vi "FITS - Make Single FITS Header.vi"(7 "Neo Info":T1={"Handle"=104, "Pixel Encoding"="Mono16", "AOI Width"=2560, "AOI Height"=2160, "AOI Stride"=5136, "Image Bytes"=11098896, "Image Pixels"=5529600, "Row Readout Time"=9.371428571428572e-06, "Frame Readout Time"=0.010121142857142858, "Interframe Time"=8.434285714285715e-05, "Semaphore"=refnum, "SerialNumber"="SCC-02209", "Camera Model"="DC-152Q-C00-FI", "Controller ID"="3", "Firmware Version"="13.8.26.122", "Shutter"="Global", "Binning"=0, "Time at Synch"=timestamp(3029526000.379448 s since 1904-01-01), "Idx"=0} {"Time at Synch" format="%<%H:%M:%S>T"; "Interframe Time" format="%#_3g"; "Frame Readout Time" format="%_3g"; "Row Readout Time" format="%_3g"}, 8 "error in":errorcluster, 9 "NAXIS":string="2", 10 "FITS Header":T3={"Wavelength (nm)"=530.15, "Exposure (s)"=0.05, "Tuning Delay (ms)"=1000.0, "Beam Type (-1/1)"=1.0, "Tuning Voltages"=[1.111, 2.222, 3.333, 4.444], "Observer"="observer", "Light Shapping Diffuser"=enum."In Beam", "Comment"="", "Data Type"=9, "Mod Cycles"=0, "SCD Calibration Optics"=enum."1 - Polarizer @0, I+Q", "SCD Emission Line Filter"=enum."1-557.6nm", "Cookbook"="", "COMP-S Calibration Wheel"=enum."Dark", "COMP-S Andover Filter Wheel"=enum."530.3nm/HWB 0.34nm (Fe XIV)", "FOV Rotation (deg)"=66.0, "Objective Lens Position (mm)"=0.0, "Occulter size"=0.0, "Time End"=timestamp(3382374145.421875 s since 1904-01-01), "Acc Exposure (s)"=0.0, "Time Stamp Array"=[], "Camera Serial Number"=[], "Camera Temp"=[], "Camera PI (mm)"=[0.0, 0.0, 0.0], "Time Start"=timestamp(3382374145.421875 s since 1904-01-01), "Peripherals"={"ILX controler"=FALSE, "Zone temperatures"=FALSE, "Andor"=FALSE, "Andor 2"=FALSE, "PI Stages"=FALSE, "AISAS mechanisms"=FALSE, "AISAS Mech.lvclass"=refnum, "Zone temp ref"=variant, "FWs"=FALSE}, "FITS paths"=[path " ", path " ", path " ", path " "], "Cameras"=enum."Andor", "load preset cbk"=FALSE, "periodic check count"=0} {"Camera PI (mm)" format="%_3g"; "Acc Exposure (s)" format="%^.3g"; "Occulter size" format="%.2f"; "Objective Lens Position (mm)" min=70.0 max=152.0 format="%.2f"; "FOV Rotation (deg)" format="%.1f"; "Data Type" items=["LIVE", "DARK", "FLAT", "CALI", "OBSE", "ABSO", "AURE", "TARG", "OBJE", "HOLE", "OREX", "THRO", "CHIP"]; "Exposure (s)" format="%^.3g"; "Wavelength (nm)" format="%_6g"}, 11 "Image #":i32) -> (0 "error out":errorcluster, 1 "23040 Byte Header":string="SIMPLE  =                              T / CONFORMS TO FITS STANDARD            BITPIX  =                             32 / BITS PER PIXEL                       NAXIS   =                              2 / DATA DIMENSIONS IN FITS FILE         NAXIS1  =                              0 / XDIM (PIXELS)                        NAXIS2  =                              0 / YDIM (PIXELS)                        NAXIS3  =                              4 / 4 POLARIZATION STATES                NAXIS4  =                              1 / 1 CAMERA                             ORIGIN  =                        'AISAS' / SCIENTIFIC GROUP                     OBSERVER=                     'SCHWARTZ' / NAME OF OBSERVER                     TELESCOP=                   '20CM ZEISS' / NAME OF TELESCOPE                    LOCATION=            'LOMNICKY PEAK OBS' / LOCATION OF TELESCOPE                INSTRUME=                          'SCD' / NAME OF INSTRUMENT                   BZERO   =                             0. /  ADU OFFSET                          FOCUS   =                             26 / CAMERA-STAGE POSITION (MM)           ROTPOS  =                           66.0 / ROTATIONAL POSITION (DEG)            DIFFUSER=                      'IN BEAM' / 0=IN BEAM, 1=OUT OF BEAM             FW-WVLNG=                        '557.6' / PRE-FILTER CENTER WAVELENGTH (NM)    FW-CALIB=                         'DARK' / CAL-WHEEL POSITION                   CAM-SN1 =                    'SCC-02209' / CAMERA SERIAL NUMBER                 CAM-TEMP=                       0.000000 / FOCAL PLANE TEMP (C)                 TUNEDLAY=                           1000 / LCVR RELAXATION DELAY (mS)           DATE_OBS=                     '3/7/2011' / DATE OF OBSERVATION START (UTC)      TIME_OBS=                   '212225.421' / TIME OF OBSERVATION (UTC)            EXPOSURE=                       0.050000 / EXPOSURE TIME (S)                    MODC    =                              0 / NUMBER OF IMAGES AT EACH STATE       NLC-1   =                          1.111 / TUNING VOLTAGE-1                     NLC-2   =                          2.222 / TUNING VOLTAGE-2                     NLC-3   =                          3.333 / TUNING VOLTAGE-3                     NLC-4   =                          4.444 / TUNING VOLTAGE-4                     NLC-5   =                          0.000 / TUNING VOLTAGE-5                     BEAM    =                              1 / BEAM (0=ON BAND OR 1=CONTINUUM)      WAVELENG=                         530.15 / WAVELENGTH OF OBS (NM)               COMMHEAD=                             '' / OBSERVER COMMENT                     COOKBOOK=                                / COOKBOOK  LOADED                     COMMENT                                                                         COMMENT                                                                         COMMENT                                                                         COMMENT                                                                         COMMENT                                                                         COMMENT                                                                         COMMENT                                                                         COMMENT                                                                         COMMENT                                                                         COMMENT                                                                         COMMENT                                                                         COMMENT                                                                         COMMENT                                                                         COMMENT                                                                         COMMENT                                                                         COMMENT                                                                         COMMENT                                                                         COMMENT                                                                         COMMENT                                                                         COMMENT                                                                         COMMENT                                                                         COMMENT                                                                         COMMENT                                                                         COMMENT                                                                         COMMENT                                                                         COMMENT                                                                         COMMENT                                                                         COMMENT                                                                         COMMENT                                                                         COMMENT                                                                         COMMENT                                                                         COMMENT                                                                         COMMENT                                                                         COMMENT                                                                         COMMENT                                                                         COMMENT                                                                         COMMENT                                                                         COMMENT                                                                         COMMENT                                                                         COMMENT                                                                         COMMENT                                                                         COMMENT                                                                         COMMENT                                                                         COMMENT                                                                         COMMENT                                                                         COMMENT                                                                         COMMENT                                                                         COMMENT                                                                         COMMENT                                                                         COMMENT                                                                         COMMENT                                                                         COMMENT                                                                         COMMENT                                                                         COMMENT                                                                         COMMENT                                                                         COMMENT                                                                         COMMENT                                                                         COMMENT                                                                         COMMENT                                                                         COMMENT                                                                         COMMENT                                                                         COMMENT                                                                         COMMENT                                                                         COMMENT                                                                         COMMENT                                                                         COMMENT                                                                         COMMENT                                                                         COMMENT                                                                         COMMENT                                                                         COMMENT                                                                         COMMENT                                                                         COMMENT                                                                         COMMENT                                                                         COMMENT                                                                         COMMENT                                                                         COMMENT                                                                         COMMENT                                                                         COMMENT                                                                         COMMENT                                                                         COMMENT                                                                         COMMENT                                                                         COMMENT                                                                         COMMENT                                                                         COMMENT                                                                         COMMENT                                                                         COMMENT                                                                         COMMENT                                                                         COMMENT                                                                         COMMENT                                                                         COMMENT                                                                         COMMENT                                                                         COMMENT                                                                         COMMENT                                                                         COMMENT                                                                         COMMENT                                                                         COMMENT                                                                         COMMENT                                                                         COMMENT                                                                         COMMENT                                                                         COMMENT                                                                         COMMENT                                                                         COMMENT                                                                         COMMENT                                                                         COMMENT                                                                         COMMENT                                                                         COMMENT                                                                         COMMENT                                                                         COMMENT                                                                         COMMENT                                                                         COMMENT                                                                         COMMENT                                                                         COMMENT                                                                         COMMENT                                                                         COMMENT                                                                         COMMENT                                                                         COMMENT                                                                         COMMENT                                                                         COMMENT                                                                         COMMENT                                                                         COMMENT                                                                         COMMENT                                                                         COMMENT                                                                         COMMENT                                                                         COMMENT                                                                         COMMENT                                                                         COMMENT                                                                         COMMENT                                                                         COMMENT                                                                         COMMENT                                                                         COMMENT                                                                         COMMENT                                                                         COMMENT                                                                         COMMENT                                                                         COMMENT                                                                         COMMENT                                                                         COMMENT                                                                         COMMENT                                                                         COMMENT                                                                         COMMENT                                                                         COMMENT                                                                         COMMENT                                                                         COMMENT                                                                         COMMENT                                                                         COMMENT                                                                         COMMENT                                                                         COMMENT                                                                         COMMENT                                                                         COMMENT                                                                         COMMENT                                                                         COMMENT                                                                         COMMENT                                                                         COMMENT                                                                         COMMENT                                                                         COMMENT                                                                         COMMENT                                                                         COMMENT                                                                         COMMENT                                                                         COMMENT                                                                         COMMENT                                                                         COMMENT                                                                         COMMENT                                                                         COMMENT                                                                         COMMENT                                                                         COMMENT                                                                         COMMENT                                                                         COMMENT                                                                         COMMENT                                                                         COMMENT                                                                         COMMENT                                                                         COMMENT                                                                         COMMENT                                                                         COMMENT                                                                         COMMENT                                                                         COMMENT                                                                         COMMENT                                                                         COMMENT                                                                         COMMENT                                                                         COMMENT                                                                         COMMENT                                                                         COMMENT                                                                         COMMENT                                                                         COMMENT                                                                         COMMENT                                                                         COMMENT                                                                         COMMENT                                                                         COMMENT                                                                         COMMENT                                                                         COMMENT                                                                         COMMENT                                                                         COMMENT                                                                         COMMENT                                                                         COMMENT                                                                         COMMENT                                                                         COMMENT                                                                         COMMENT                                                                         COMMENT                                                                         COMMENT                                                                         COMMENT                                                                         COMMENT                                                                         COMMENT                                                                         COMMENT                                                                         COMMENT                                                                         COMMENT                                                                         COMMENT                                                                         COMMENT                                                                         COMMENT                                                                         COMMENT                                                                         COMMENT                                                                         COMMENT                                                                         COMMENT                                                                         COMMENT                                                                         COMMENT                                                                         COMMENT                                                                         COMMENT                                                                         COMMENT                                                                         COMMENT                                                                         COMMENT                                                                         COMMENT                                                                         COMMENT                                                                         COMMENT                                                                         COMMENT                                                                         COMMENT                                                                         COMMENT                                                                         COMMENT                                                                         COMMENT                                                                         COMMENT                                                                         COMMENT                                                                         COMMENT                                                                         COMMENT                                                                         COMMENT                                                                         COMMENT                                                                         COMMENT                                                                         COMMENT                                                                         COMMENT                                                                         COMMENT                                                                         COMMENT                                                                         COMMENT                                                                         COMMENT                                                                         COMMENT                                                                         COMMENT                                                                         COMMENT                                                                         COMMENT                                                                         COMMENT                                                                         COMMENT                                                                         COMMENT                                                                         COMMENT                                                                         COMMENT                                                                         COMMENT                                                                         COMMENT                                                                         COMMENT                                                                         COMMENT                                                                         COMMENT                                                                         COMMENT                                                                         END                                                                             ", 3 "final header byte length":i32=23040)   [LabVIEW 2014]
uses:
  Controls/SCD - Calibration Optics Filter Wheel.ctl
  AISAS/Controls/Diffuser.ctl
  Controls/SCD - FITS Cluster.ctl
  Controls/SCD - EDT - Emission Line Filter Wheel.ctl
  Camera/Andor Neo Info.ctl
  Controls/CoMP-S Controls/Polarization Optics Filter Wheel.ctl
  Controls/CoMP-S Controls/Emission Line Filter Wheel.ctl
  AISAS/Controls/focus.ctl
  AISAS/Mech/AISAS Mech.lvclass
  Controls/peripherals.ctl
  Controls/Cameras select.ctl
panel:
  out "Required COMMENT Rows":i32
  in  "BITPIX":string="32"
  in  "BZERO":string="0."
  in  "NAXIS2":string="2160"
  in  "NAXIS1":string="2560"
  out "Header Rows":i32=34
  out "FITS Header":string[](array[string])=["SIMPLE  =                              T / CONFORMS TO FITS STANDARD            ", "BITPIX  =                             32 / BITS PER PIXEL                       ", "NAXIS   =                              2 / DATA DIMENSIONS IN FITS FILE         ", "NAXIS1  =                              0 / XDIM (PIXELS)                        ", "NAXIS2  =                              0 / YDIM (PIXELS)                        ", "NAXIS3  =                              4 / 4 POLARIZATION STATES                ", "NAXIS4  =                              1 / 1 CAMERA                             ", "ORIGIN  =                        'AISAS' / SCIENTIFIC GROUP                     ", "OBSERVER=                     'SCHWARTZ' / NAME OF OBSERVER                     ", "TELESCOP=                   '20CM ZEISS' / NAME OF TELESCOPE                    ", "LOCATION=            'LOMNICKY PEAK OBS' / LOCATION OF TELESCOPE                ", "INSTRUME=                          'SCD' / NAME OF INSTRUMENT                   ", "BZERO   =                             0. /  ADU OFFSET                          ", "FOCUS   =                             26 / CAMERA-STAGE POSITION (MM)           ", "ROTPOS  =                           66.0 / ROTATIONAL POSITION (DEG)            ", "DIFFUSER=                      'IN BEAM' / 0=IN BEAM, 1=OUT OF BEAM             ", "FW-WVLNG=                        '557.6' / PRE-FILTER CENTER WAVELENGTH (NM)    ", "FW-CALIB=                         'DARK' / CAL-WHEEL POSITION                   ", "CAM-SN1 =                    'SCC-02209' / CAMERA SERIAL NUMBER                 ", "CAM-TEMP=                       0.000000 / FOCAL PLANE TEMP (C)                 ", "TUNEDLAY=                           1000 / LCVR RELAXATION DELAY (mS)           ", "DATE_OBS=                     '3/7/2011' / DATE OF OBSERVATION START (UTC)      ", "TIME_OBS=                   '212225.421' / TIME OF OBSERVATION (UTC)            ", "EXPOSURE=                       0.050000 / EXPOSURE TIME (S)                    ", "MODC    =                              0 / NUMBER OF IMAGES AT EACH STATE       ", "NLC-1   =                          1.111 / TUNING VOLTAGE-1                     ", "NLC-2   =                          2.222 / TUNING VOLTAGE-2                     ", "NLC-3   =                          3.333 / TUNING VOLTAGE-3                     ", "NLC-4   =                          4.444 / TUNING VOLTAGE-4                     ", "NLC-5   =                          0.000 / TUNING VOLTAGE-5                     ", "BEAM    =                              1 / BEAM (0=ON BAND OR 1=CONTINUUM)      ", "WAVELENG=                         530.15 / WAVELENGTH OF OBS (NM)               ", "COMMHEAD=                             '' / OBSERVER COMMENT                     ", "COOKBOOK=                                / COOKBOOK  LOADED                     ", "COMMENT                                                                         ", "COMMENT                                                                         ", "COMMENT                                                                         ", "COMMENT                                                                         ", "COMMENT                                                                         ", "COMMENT                                                                         ", "COMMENT                                                                         ", "COMMENT                                                                         ", "COMMENT                                                                         ", "COMMENT                                                                         ", "COMMENT                                                                         ", "COMMENT                                                                         ", "COMMENT                                                                         ", "COMMENT                                                                         ", "COMMENT                                                                         ", "COMMENT                                                                         ", "COMMENT                                                                         ", "COMMENT                                                                         ", "COMMENT                                                                         ", "COMMENT                                                                         ", "COMMENT                                                                         ", "COMMENT                                                                         ", "COMMENT                                                                         ", "COMMENT                                                                         ", "COMMENT                                                                         ", "COMMENT                                                                         ", "COMMENT                                                                         ", "COMMENT                                                                         ", "COMMENT                                                                         ", "COMMENT                                                                         ", "COMMENT                                                                         ", "COMMENT                                                                         ", "COMMENT                                                                         ", "COMMENT                                                                         ", "COMMENT                                                                         ", "COMMENT                                                                         ", "COMMENT                                                                         ", "COMMENT                                                                         ", "COMMENT                                                                         ", "COMMENT                                                                         ", "COMMENT                                                                         ", "COMMENT                                                                         ", "COMMENT                                                                         ", "COMMENT                                                                         ", "COMMENT                                                                         ", "COMMENT                                                                         ", "COMMENT                                                                         ", "COMMENT                                                                         ", "COMMENT                                                                         ", "COMMENT                                                                         ", "COMMENT                                                                         ", "COMMENT                                                                         ", "COMMENT                                                                         ", "COMMENT                                                                         ", "COMMENT                                                                         ", "COMMENT                                                                         ", "COMMENT                                                                         ", "COMMENT                                                                         ", "COMMENT                                                                         ", "COMMENT                                                                         ", "COMMENT                                                                         ", "COMMENT                                                                         ", "COMMENT                                                                         ", "COMMENT                                                                         ", "COMMENT                                                                         ", "COMMENT                                                                         ", "COMMENT                                                                         ", "COMMENT                                                                         ", "COMMENT                                                                         ", "COMMENT                                                                         ", "COMMENT                                                                         ", "COMMENT                                                                         ", "COMMENT                                                                         ", "COMMENT                                                                         ", "COMMENT                                                                         ", "COMMENT                                                                         ", "COMMENT                                                                         ", "COMMENT                                                                         ", "COMMENT                                                                         ", "COMMENT                                                                         ", "COMMENT                                                                         ", "COMMENT                                                                         ", "COMMENT                                                                         ", "COMMENT                                                                         ", "COMMENT                                                                         ", "COMMENT                                                                         ", "COMMENT                                                                         ", "COMMENT                                                                         ", "COMMENT                                                                         ", "COMMENT                                                                         ", "COMMENT                                                                         ", "COMMENT                                                                         ", "COMMENT                                                                         ", "COMMENT                                                                         ", "COMMENT                                                                         ", "COMMENT                                                                         ", "COMMENT                                                                         ", "COMMENT                                                                         ", "COMMENT                                                                         ", "COMMENT                                                                         ", "COMMENT                                                                         ", "COMMENT                                                                         ", "COMMENT                                                                         ", "COMMENT                                                                         ", "COMMENT                                                                         ", "COMMENT                                                                         ", "COMMENT                                                                         ", "COMMENT                                                                         ", "COMMENT                                                                         ", "COMMENT                                                                         ", "COMMENT                                                                         ", "COMMENT                                                                         ", "COMMENT                                                                         ", "COMMENT                                                                         ", "COMMENT                                                                         ", "COMMENT                                                                         ", "COMMENT                                                                         ", "COMMENT                                                                         ", "COMMENT                                                                         ", "COMMENT                                                                         ", "COMMENT                                                                         ", "COMMENT                                                                         ", "COMMENT                                                                         ", "COMMENT                                                                         ", "COMMENT                                                                         ", "COMMENT                                                                         ", "COMMENT                                                                         ", "COMMENT                                                                         ", "COMMENT                                                                         ", "COMMENT                                                                         ", "COMMENT                                                                         ", "COMMENT                                                                         ", "COMMENT                                                                         ", "COMMENT                                                                         ", "COMMENT                                                                         ", "COMMENT                                                                         ", "COMMENT                                                                         ", "COMMENT                                                                         ", "COMMENT                                                                         ", "COMMENT                                                                         ", "COMMENT                                                                         ", "COMMENT                                                                         ", "COMMENT                                                                         ", "COMMENT                                                                         ", "COMMENT                                                                         ", "COMMENT                                                                         ", "COMMENT                                                                         ", "COMMENT                                                                         ", "COMMENT                                                                         ", "COMMENT                                                                         ", "COMMENT                                                                         ", "COMMENT                                                                         ", "COMMENT                                                                         ", "COMMENT                                                                         ", "COMMENT                                                                         ", "COMMENT                                                                         ", "COMMENT                                                                         ", "COMMENT                                                                         ", "COMMENT                                                                         ", "COMMENT                                                                         ", "COMMENT                                                                         ", "COMMENT                                                                         ", "COMMENT                                                                         ", "COMMENT                                                                         ", "COMMENT                                                                         ", "COMMENT                                                                         ", "COMMENT                                                                         ", "COMMENT                                                                         ", "COMMENT                                                                         ", "COMMENT                                                                         ", "COMMENT                                                                         ", "COMMENT                                                                         ", "COMMENT                                                                         ", "COMMENT                                                                         ", "COMMENT                                                                         ", "COMMENT                                                                         ", "COMMENT                                                                         ", "COMMENT                                                                         ", "COMMENT                                                                         ", "COMMENT                                                                         ", "COMMENT                                                                         ", "COMMENT                                                                         ", "COMMENT                                                                         ", "COMMENT                                                                         ", "COMMENT                                                                         ", "COMMENT                                                                         ", "COMMENT                                                                         ", "COMMENT                                                                         ", "COMMENT                                                                         ", "COMMENT                                                                         ", "COMMENT                                                                         ", "COMMENT                                                                         ", "COMMENT                                                                         ", "COMMENT                                                                         ", "COMMENT                                                                         ", "COMMENT                                                                         ", "COMMENT                                                                         ", "COMMENT                                                                         ", "COMMENT                                                                         ", "COMMENT                                                                         ", "COMMENT                                                                         ", "COMMENT                                                                         ", "COMMENT                                                                         ", "COMMENT                                                                         ", "COMMENT                                                                         ", "COMMENT                                                                         ", "COMMENT                                                                         ", "COMMENT                                                                         ", "COMMENT                                                                         ", "COMMENT                                                                         ", "COMMENT                                                                         ", "COMMENT                                                                         ", "COMMENT                                                                         ", "COMMENT                                                                         ", "COMMENT                                                                         ", "COMMENT                                                                         ", "COMMENT                                                                         ", "COMMENT                                                                         ", "COMMENT                                                                         ", "COMMENT                                                                         ", "COMMENT                                                                         ", "COMMENT                                                                         ", "COMMENT                                                                         ", "COMMENT                                                                         ", "COMMENT                                                                         ", "COMMENT                                                                         ", "COMMENT                                                                         ", "COMMENT                                                                         ", "COMMENT                                                                         ", "COMMENT                                                                         ", "COMMENT                                                                         ", "COMMENT                                                                         ", "COMMENT                                                                         ", "COMMENT                                                                         ", "COMMENT                                                                         ", "COMMENT                                                                         ", "COMMENT                                                                         ", "COMMENT                                                                         ", "COMMENT                                                                         ", "COMMENT                                                                         ", "COMMENT                                                                         ", "COMMENT                                                                         ", "COMMENT                                                                         ", "COMMENT                                                                         ", "COMMENT                                                                         ", "COMMENT                                                                         ", "COMMENT                                                                         ", "COMMENT                                                                         ", "COMMENT                                                                         ", "COMMENT                                                                         ", "COMMENT                                                                         ", "COMMENT                                                                         ", "COMMENT                                                                         ", "END                                                                             "]
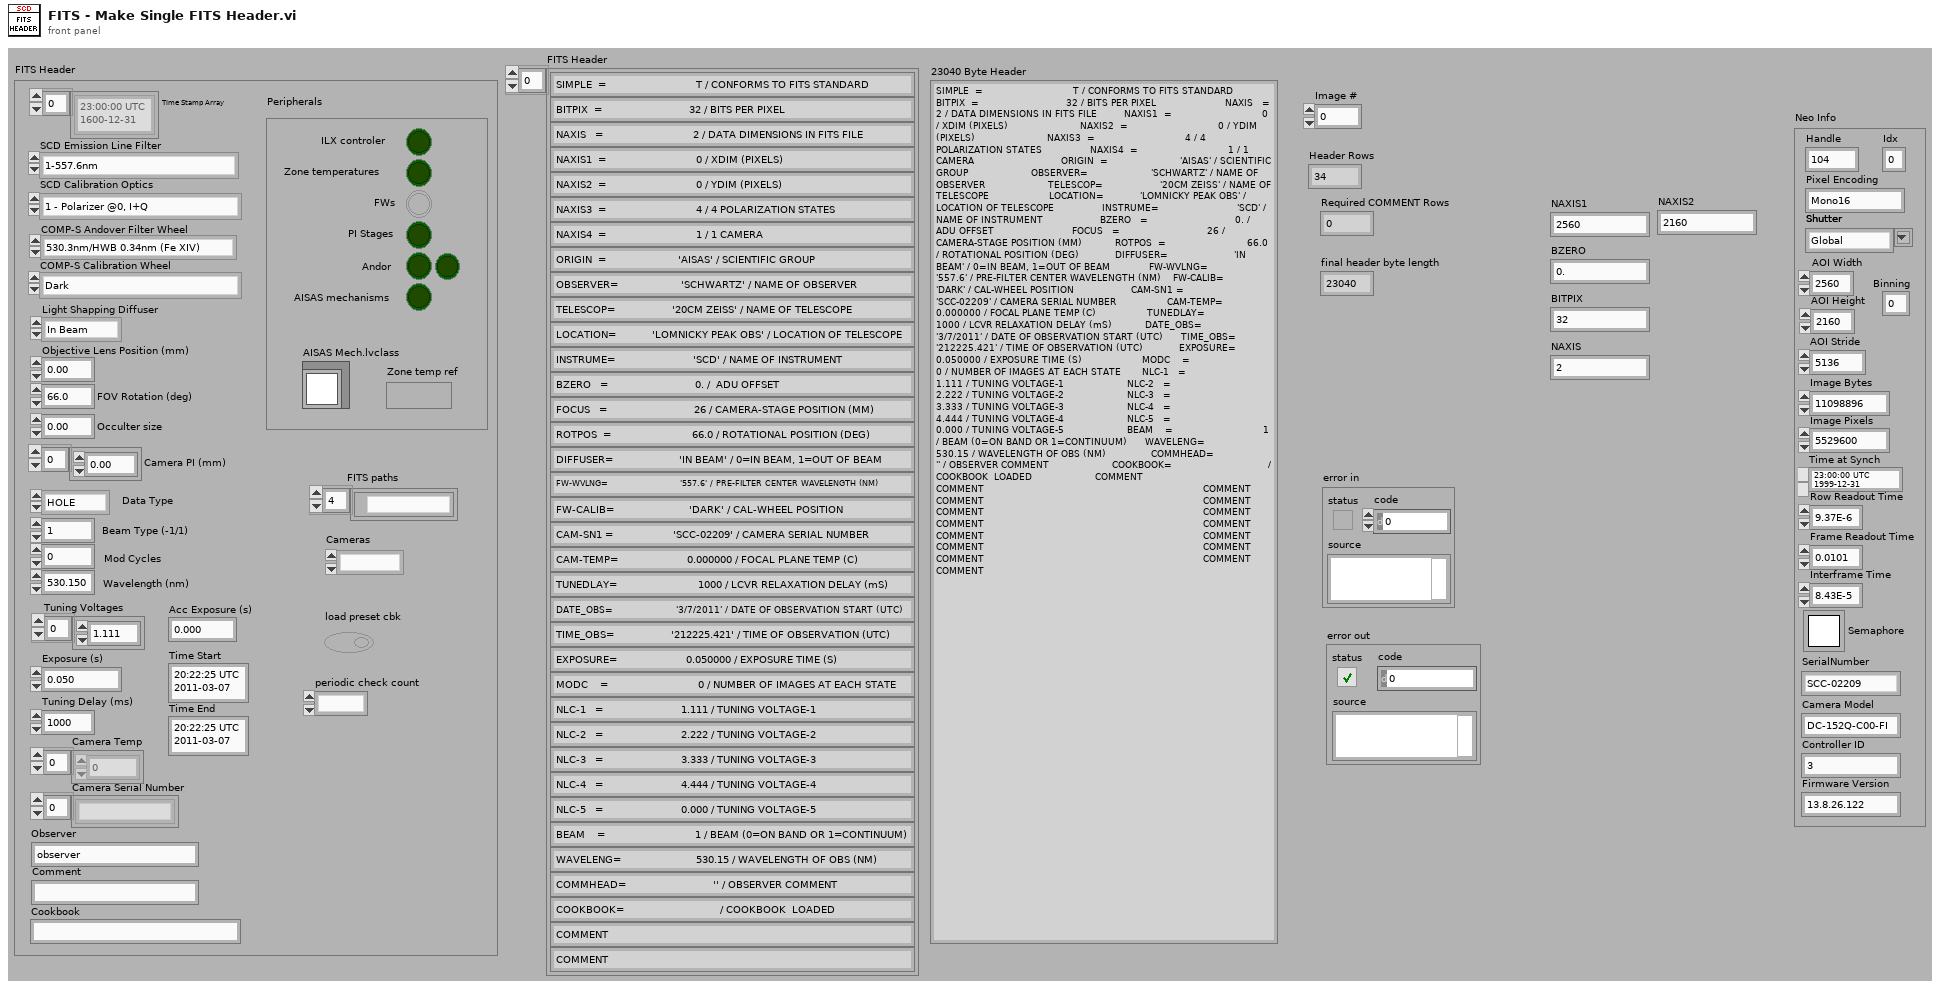
[diagram p1: front panel]
types:
  T1 = typedef "Andor Neo Info.ctl" = cluster{"Handle":i32, "Pixel Encoding":string, "AOI Width":i64, "AOI Height":i64, "AOI Stride":i64, "Image Bytes":i64, "Image Pixels":i64, "Row Readout Time":dbl, "Frame Readout Time":dbl, "Interframe Time":dbl, "Semaphore":T2, "SerialNumber":string, "Camera Model":string, "Controller ID":string, "Firmware Version":string, "Shutter":string, "Binning":u8, "Time at Synch":timestamp, "Idx":i32}
  T2 = typedef "Semaphore RefNum" = refnum<k1>
  T3 = typedef "SCD - FITS Cluster.ctl" = cluster{"Wavelength (nm)":dbl, "Exposure (s)":dbl, "Tuning Delay (ms)":dbl, "Beam Type (-1/1)":dbl, "Tuning Voltages":dbl[], "Observer":string, "Light Shapping Diffuser":T4, "Comment":string, "Data Type":u16, "Mod Cycles":u16, "SCD Calibration Optics":T5, "SCD Emission Line Filter":T6, "Cookbook":string, "COMP-S Calibration Wheel":T7, "COMP-S Andover Filter Wheel":T8, "FOV Rotation (deg)":dbl, "Objective Lens Position (mm)":T9, "Occulter size":dbl, "Time End":timestamp, "Acc Exposure (s)":dbl, "Time Stamp Array":timestamp[], "Camera Serial Number":string[], "Camera Temp":dbl[], "Camera PI (mm)":dbl[], "Time Start":timestamp, "Peripherals":T10, "FITS paths":path[], "Cameras":T11, "load preset cbk":bool, "periodic check count":i32}
  T4 = typedef "Diffuser.ctl" = enum16{"Out of Beam", "In Beam"}
  T5 = typedef "SCD - Calibration Optics Filter Wheel.ctl" = enum16{"1 - Polarizer @0, I+Q", "2 - Polarizer @90, I-Q", "3 - Polarizer @45, I+U", "4 - Polarizer @135, I-U", "5 - Polarizer @0, Retarder @45, I+V", "6 - Polarizer @0, Retarder @135, I-V", "7 - Dark", "8 - Clear", "9 - N/A"}
  T6 = typedef "SCD - EDT - Emission Line Filter Wheel.ctl" = enum16{"1-557.6nm", "2-587.6nm", "3-589.6nm", "4-630.2nm", "5-656.4nm", "6-849.8nm", "7-854.2nm", "8-866.2nm", "9-1083.0nm"}
  T7 = typedef "Polarization Optics Filter Wheel.ctl" = enum16{"Dark", "Clear", "Exchange Lens", "Polarizer @0, I+Q", "Polarizer @90, I-Q", "Polarizer @45, I+U", "Polarizer @135, I-U", "Polarizer @0, Retarder @45, I+V", "Polarizer @0, Retarder @135, I-V"}
  T8 = typedef "Emission Line Filter Wheel.ctl" = enum16{"530.3nm/HWB 0.34nm (Fe XIV)", "587.6nm/HBW 0.44nm (He I D3)", "637.5nm/HBW 0.53nm (Fe X)", "656.3nm/HBW 0.57nm (H-Alpha)", "789.2nm/HBW 0.85nm (Fe XI)", "854.2nm/HBW 1.01nm (Ca I)", "1074.7nm/HBW 2.34nm (Fe XIII)", "1079.8nm/HBW 1.64nm (Fe XIII)", "1083.0nm/HBW 1.66nm (He I)"}
  T9 = typedef "focus.ctl" = dbl
  T10 = typedef "peripherals.ctl" = cluster{"ILX controler":bool, "Zone temperatures":bool, "Andor":bool, "Andor 2":bool, "PI Stages":bool, "AISAS mechanisms":bool, "AISAS Mech.lvclass":refnum<class "AISAS Mech.lvclass">, "Zone temp ref":variant, "FWs":bool}
  T11 = typedef "Cameras select.ctl" = enum16{"Andor", "GDR"}
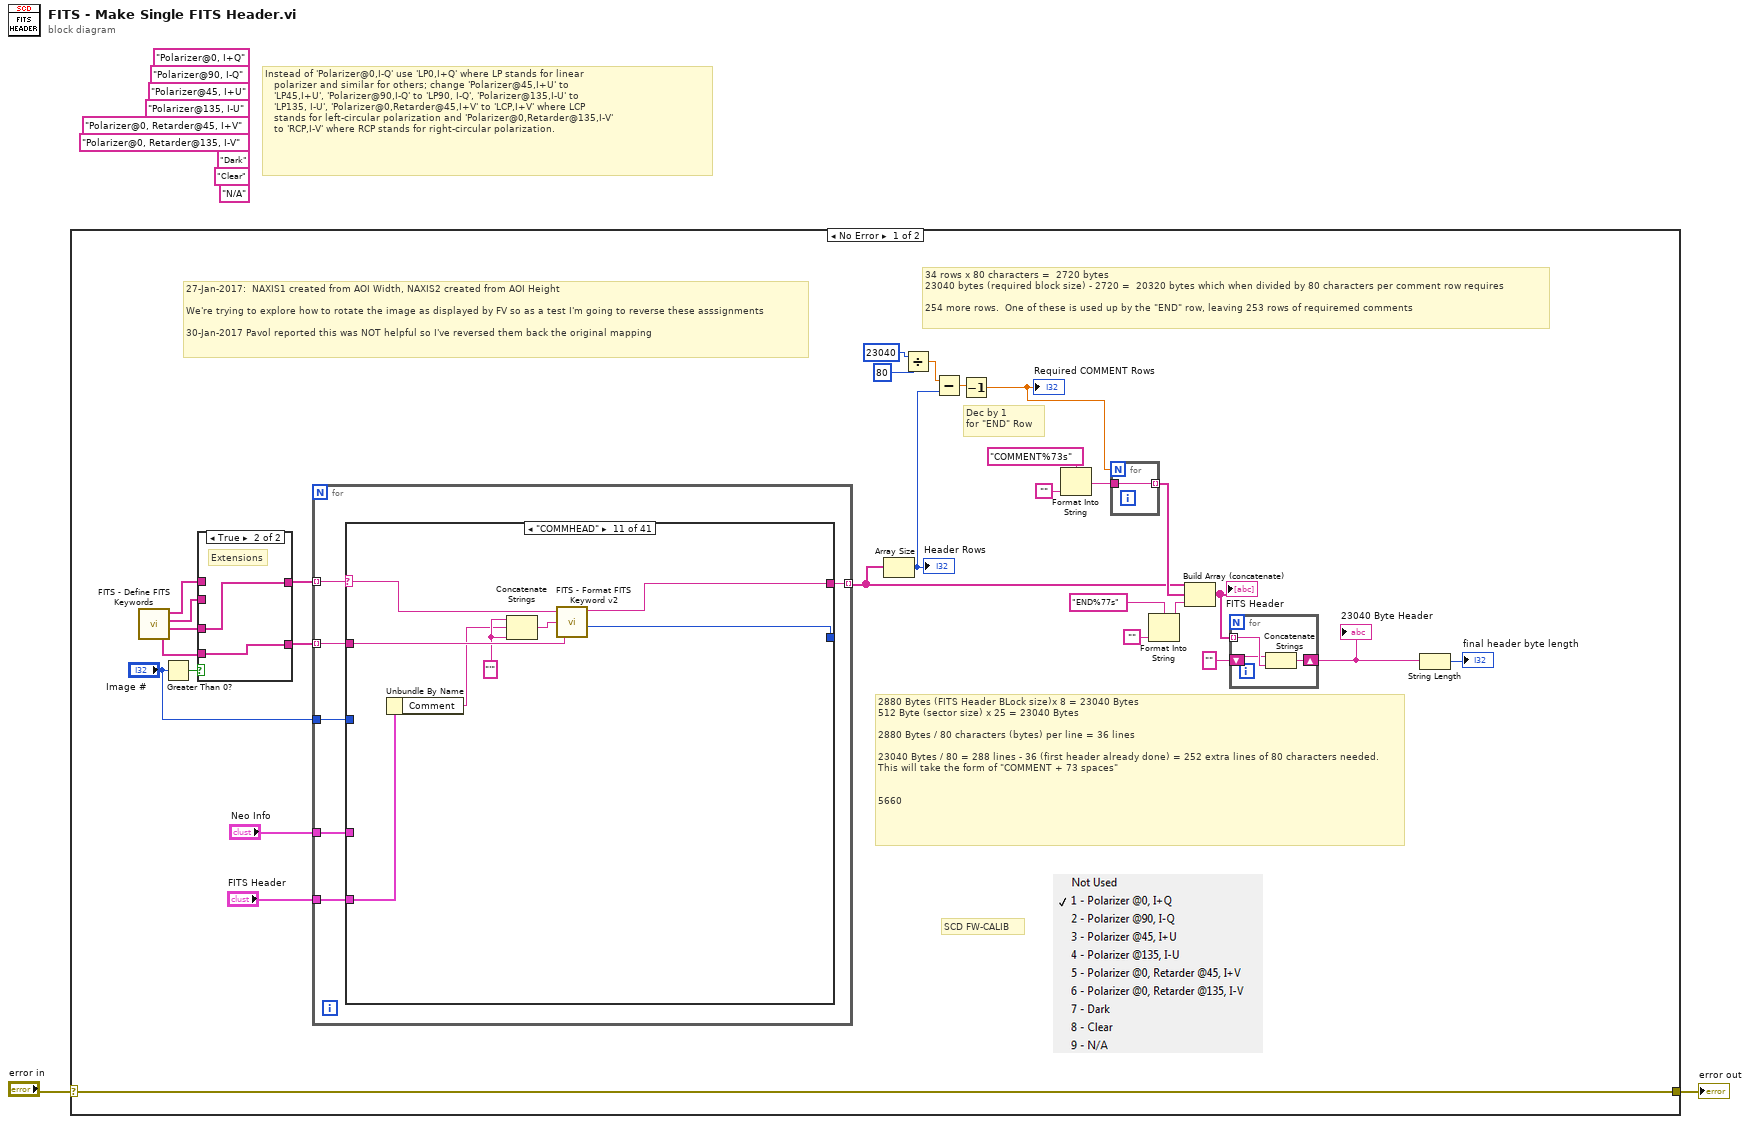
[diagram p0: block diagram]
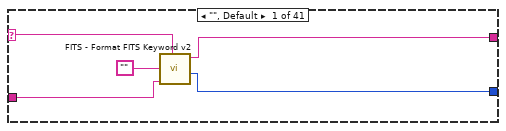
[diagram p3: hidden frame]
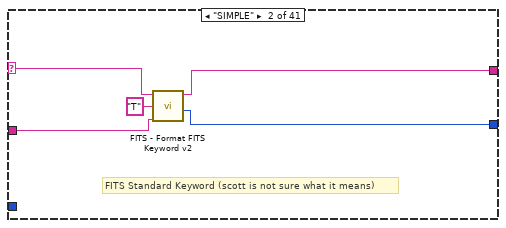
[diagram p4: hidden frame]
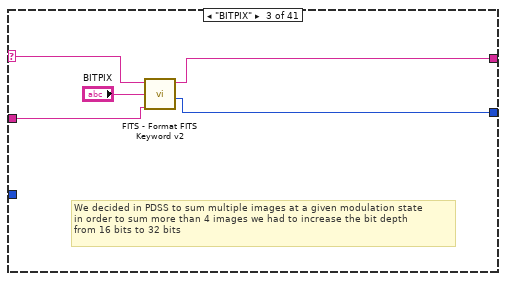
[diagram p5: hidden frame]
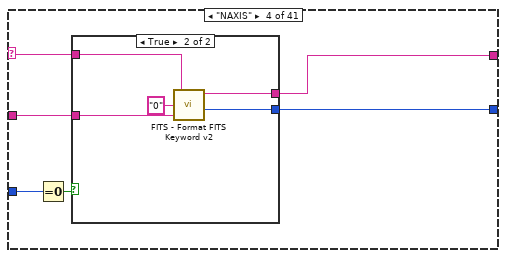
[diagram p6: hidden frame]
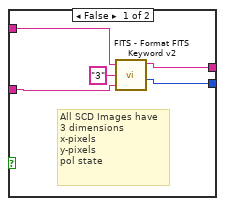
[diagram p7: hidden frame]
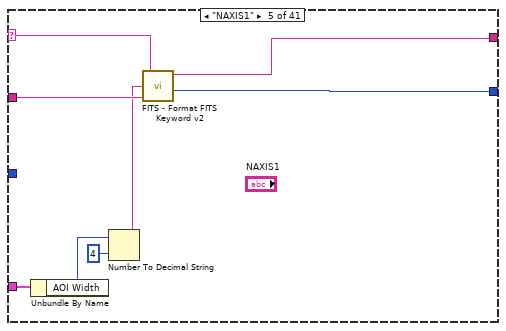
[diagram p8: hidden frame]
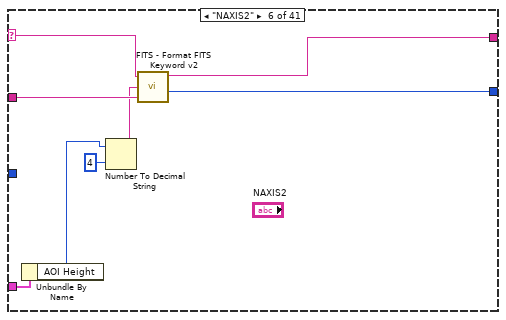
[diagram p9: hidden frame]
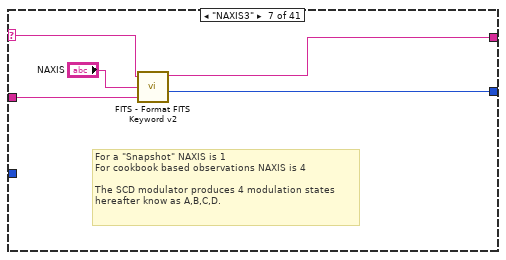
[diagram p10: hidden frame]
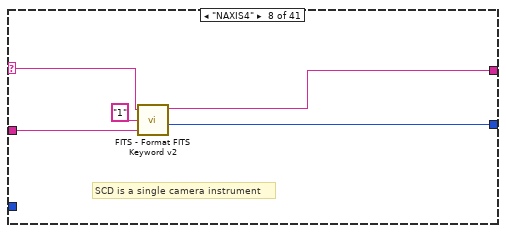
[diagram p11: hidden frame]
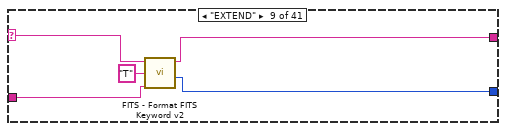
[diagram p12: hidden frame]
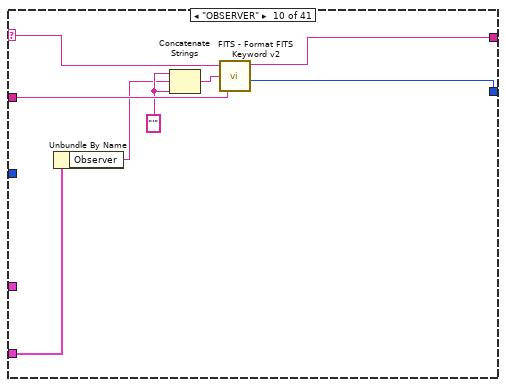
[diagram p13: hidden frame]
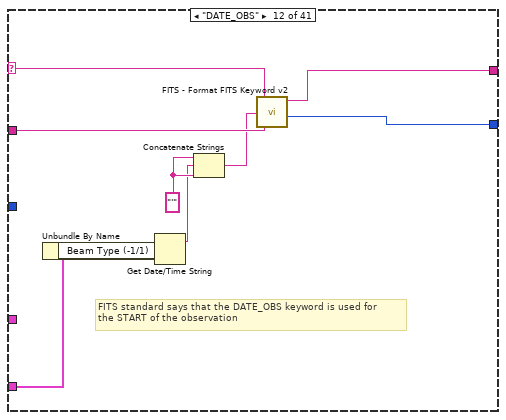
[diagram p14: hidden frame]
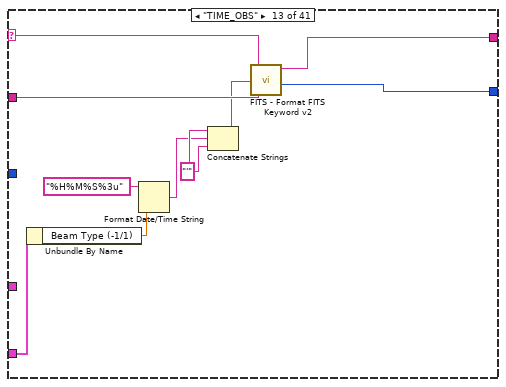
[diagram p15: hidden frame]
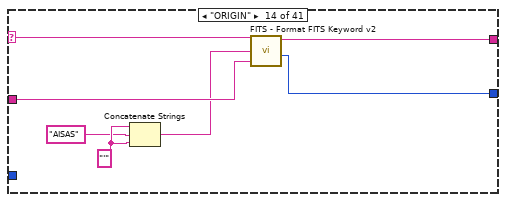
[diagram p16: hidden frame]
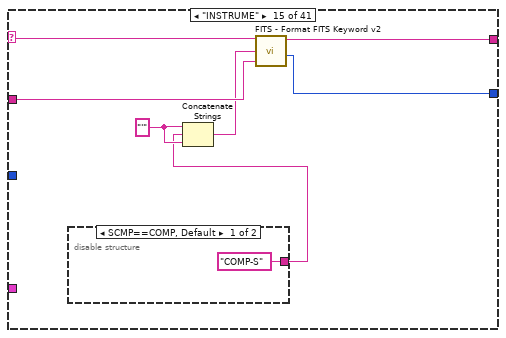
[diagram p17: hidden frame]
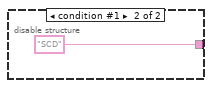
[diagram p18: hidden frame]
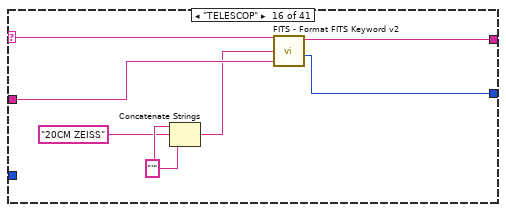
[diagram p19: hidden frame]
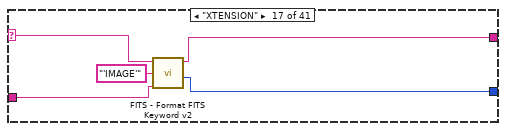
[diagram p20: hidden frame]
diagram:
  (unwired) "N/A" ("element")
  (unwired) "Clear" ("element")
  (unwired) "Dark" ("element")
  (unwired) "Polarizer@0, Retarder@135, I-V" ("element")
  (unwired) "Polarizer@0, Retarder@45, I+V" ("element")
  (unwired) "Polarizer@135, I-U" ("element")
  (unwired) "Polarizer@45, I+U"
  (unwired) "Polarizer@90, I-Q"
  (unwired) "Polarizer@0, I+Q"
  # "Instead of 'Polarizer@0,I-Q' use 'LP0,I+Q' where LP stands for linear\n   polarizer and similar for others; change 'Polarizer@45,I+U' to\n   'LP45,I+U', 'Polarizer@90,I-Q' to 'LP90, I-Q', 'Polarizer@135,I-U' to\n   'LP135, I-U', 'Polarizer@0,Retarder@45,I+V' to 'LCP,I+V' where LCP\n   stands for left-circular polarization and 'Polarizer@0,Retarder@135,I-V'\n   to 'RCP,I-V' where RCP stands for right-circular polarization."
  n1 = case shown="No Error" "error in" {
    selector: "error in" -> [w12 w423]
    tunnel: [w12 w423] -> w1
    frame No Error {
      # "SCD FW-CALIB"
      # "27-Jan-2017:  NAXIS1 created from AOI Width, NAXIS2 created from AOI Height\n\nWe're trying to explore how to rotate the image as displayed by FV so as a test I'm going to reverse these asssignments\n\n30-Jan-2017 Pavol reported this was NOT helpful so I've reversed them back the original mapping"
      # "34 rows x 80 characters =  2720 bytes\n23040 bytes (required block size) - 2720 =  20320 bytes which when divided by 80 characters per comment row requires\n\n254 more rows.  One of these is used up by the \"END\" row, leaving 253 rows of requiremed comments"
      # "Dec by 1\nfor \"END\" Row"
      # "2880 Bytes (FITS Header BLock size)x 8 = 23040 Bytes\n512 Byte (sector size) x 25 = 23040 Bytes\n\n2880 Bytes / 80 characters (bytes) per line = 36 lines\n\n23040 Bytes / 80 = 288 lines - 36 (first header already done) = 252 extra lines of 80 characters needed.\nThis will take the form of \"COMMENT + 73 spaces\" \n\n\n5660"
      n2 = call "FITS - Define FITS Keywords.vi"() -> ("Extension Comments"=w24:string[], "Extension  Keywords"=w25:string[], "Primary Comments"=w26:string[], "Primary Keywords"=w23:string[])  [unwired: 6 out]
      n3 = Greater Than 0?(x="Image #") -> (x > 0?=w29:bool)
      n4 = case shown="True" w29 {
        tunnel: [w37 w39] -> w28
        tunnel: [w36 w38] -> w27
        tunnel: w23 -> [w37 _]
        tunnel: w26 -> [w36 _]
        tunnel: w25 -> [_ w39]
        tunnel: w24 -> [_ w38]
        frame False {
          # "Primary"
        }
        frame True {
          # "Extensions"
        }
      }
      n5 = for {
        tunnel: w28 -> [w42] mode=indexing
        tunnel: w27 -> [w44] mode=indexing
        tunnel: "FITS Header" -> [w45]
        tunnel: [w43] -> w11 mode=indexing
        tunnel: "Neo Info" -> [w41]
        tunnel: "Image #" -> [w40]
        n6 = case shown="\"COMMHEAD\"" w42 {
          selector: w42 -> [w50 w55 w60 w66 w84 w92 w97 w102 w107 w115 w123 w132 w142 w149 w156 w165 w170 w175 w180 w187 w192 w201 w208 w218 w228 w238 w248 w258 w268 w276 w283 w290 w297 w309 w317 w353 w385 w394 w399 w404 w411]
          tunnel: w45 -> [_ _ _ _ _ _ _ _ _ w109 w117 w129 w139 _ _ _ _ _ _ _ w189 w198 w205 w215 w225 w235 w245 w255 w265 w273 w280 w287 w294 w306 w314 w350 w389 _ _ w405 w412]
          tunnel: w44 -> [w48 w54 w58 w65 w83 w91 w96 w101 w106 w114 w122 w131 w141 w148 w155 w164 w169 w173 w178 w182 w191 w200 w207 w217 w227 w237 w247 w257 w267 w275 w282 w289 w296 w308 w316 w352 w386 w393 w398 w403 w410]
          tunnel: [w47 w53 w57 w64 w82 w90 w95 w100 w105 w113 w121 w130 w140 w147 w154 w163 w168 w172 w177 w186 w190 w199 w206 w216 w226 w236 w246 w256 w266 w274 w281 w288 w295 w307 w315 w351 w384 w392 w397 w402 w409] -> w43
          tunnel: [w46 w51 w56 w63 w81 w89 w94 w98 w103 w110 w118 w126 w136 w143 w150 w159 w166 w171 w176 w181 w188 w196 w203 w211 w224 w234 w244 w254 w264 w272 w277 w284 w291 w305 w313 w349 w383 w391 w396 w401 w408] -> _
          tunnel: w41 -> [_ _ _ _ w78 w85 _ _ _ _ _ _ _ _ _ _ _ _ _ _ _ _ _ _ _ _ _ _ _ _ _ _ _ _ _ _ _ _ _ _ _]
          tunnel: w40 -> [_ _ _ w61 _ _ _ _ _ _ _ _ _ _ _ _ _ _ _ _ _ _ _ _ _ _ _ _ _ _ _ _ _ _ _ _ _ _ _ _ _]
          frame "", Default {
            n7 = call "FITS - Format FITS Keyword v2 .vi"("Keyword"=w50, "Value"="", "Comment"=w48) -> ("Formatted fits entry"=w47:string, "Length of line"=w46:i16)  [unwired: 1 in, 1 out]
          }
          frame "SIMPLE" {
            # "FITS Standard Keyword (scott is not sure what it means)"
            n8 = call "FITS - Format FITS Keyword v2 .vi"("Keyword"=w55, "Value"="T", "Comment"=w54) -> ("Formatted fits entry"=w53:string, "Length of line"=w51:i16)  [unwired: 1 in, 1 out]
          }
          frame "BITPIX" {
            # "We decided in PDSS to sum multiple images at a given modulation state\nin order to sum more than 4 images we had to increase the bit depth\nfrom 16 bits to 32 bits"
            n9 = call "FITS - Format FITS Keyword v2 .vi"("Keyword"=w60, "Value"="BITPIX", "Comment"=w58) -> ("Formatted fits entry"=w57:string, "Length of line"=w56:i16)  [unwired: 1 in, 1 out]
          }
          frame "NAXIS" {
            n10 = Equal To 0?(x=w61) -> (x = 0?=w62:bool)
            n11 = case shown="True" w62 {
              tunnel: w66 -> [w69 w76]
              tunnel: w65 -> [w70 w75]
              tunnel: [w68 w74] -> w64
              tunnel: [w67 w73] -> w63
              frame False {
                # "All SCD Images have\n3 dimensions\nx-pixels\ny-pixels\npol state"
                n12 = call "FITS - Format FITS Keyword v2 .vi"("Keyword"=w69, "Value"="3", "Comment"=w70) -> ("Formatted fits entry"=w68:string, "Length of line"=w67:i16)  [unwired: 1 in, 1 out]
              }
              frame True {
                n13 = call "FITS - Format FITS Keyword v2 .vi"("Keyword"=w76, "Value"="0", "Comment"=w75) -> ("Formatted fits entry"=w74:string, "Length of line"=w73:i16)  [unwired: 1 in, 1 out]
              }
            }
          }
          frame "NAXIS1" {
            n14 = Unbundle By Name(w78) -> ("AOI Width"=w77:i64)
            n15 = Number To Decimal String(number=w77, width (-)=i16 4) -> (decimal integer string=w79:string)
            n16 = call "FITS - Format FITS Keyword v2 .vi"("Keyword"=w84, "Value"=w79, "Comment"=w83) -> ("Formatted fits entry"=w82:string, "Length of line"=w81:i16)  [unwired: 1 in, 1 out]
          }
          frame "NAXIS2" {
            n17 = Unbundle By Name(w85) -> ("AOI Height"=w86:i64)
            n18 = Number To Decimal String(number=w86, width (-)=i16 4) -> (decimal integer string=w87:string)
            n19 = call "FITS - Format FITS Keyword v2 .vi"("Keyword"=w92, "Value"=w87, "Comment"=w91) -> ("Formatted fits entry"=w90:string, "Length of line"=w89:i16)  [unwired: 1 in, 1 out]
          }
          frame "NAXIS3" {
            # "For a \"Snapshot\" NAXIS is 1\nFor cookbook based observations NAXIS is 4\n\nThe SCD modulator produces 4 modulation states\nhereafter know as A,B,C,D."
            n20 = call "FITS - Format FITS Keyword v2 .vi"("Keyword"=w97, "Value"="NAXIS", "Comment"=w96) -> ("Formatted fits entry"=w95:string, "Length of line"=w94:i16)  [unwired: 1 in, 1 out]
          }
          frame "NAXIS4" {
            # "SCD is a single camera instrument"
            n21 = call "FITS - Format FITS Keyword v2 .vi"("Keyword"=w102, "Value"="1", "Comment"=w101) -> ("Formatted fits entry"=w100:string, "Length of line"=w98:i16)  [unwired: 1 in, 1 out]
          }
          frame "EXTEND" {
            n22 = call "FITS - Format FITS Keyword v2 .vi"("Keyword"=w107, "Value"="T", "Comment"=w106) -> ("Formatted fits entry"=w105:string, "Length of line"=w103:i16)  [unwired: 1 in, 1 out]
          }
          frame "OBSERVER" {
            w112 = "'" ("string")
            n23 = Unbundle By Name(w109) -> ("Observer"=w108:string)
            n24 = Concatenate Strings(w112, w108, w112) -> (w111:string)
            n25 = call "FITS - Format FITS Keyword v2 .vi"("Keyword"=w115, "Value"=w111, "Comment"=w114) -> ("Formatted fits entry"=w113:string, "Length of line"=w110:i16)  [unwired: 1 in, 1 out]
          }
          frame "COMMHEAD" {
            w120 = "'" ("string")
            n26 = Unbundle By Name(w117) -> ("Comment"=w116:string)
            n27 = Concatenate Strings(w120, w116, w120) -> (w119:string)
            n28 = call "FITS - Format FITS Keyword v2 .vi"("Keyword"=w123, "Value"=w119, "Comment"=w122) -> ("Formatted fits entry"=w121:string, "Length of line"=w118:i16)  [unwired: 1 in, 1 out]
          }
          frame "DATE_OBS" {
            w128 = "'" ("string")
            # "FITS standard says that the DATE_OBS keyword is used for \nthe START of the observation"
            n29 = Unbundle By Name(w129) -> ("Beam Type (-1/1)"=w125:dbl)
            n30 = Get Date/Time String(seconds (now)=w125) -> (date string=w124:string)  [unwired: 2 in, 1 out]
            n31 = Concatenate Strings(w128, w124, w128) -> (w127:string)
            n32 = call "FITS - Format FITS Keyword v2 .vi"("Keyword"=w132, "Value"=w127, "Comment"=w131) -> ("Formatted fits entry"=w130:string, "Length of line"=w126:i16)  [unwired: 1 in, 1 out]
          }
          frame "TIME_OBS" {
            w138 = "'" ("string")
            n33 = Unbundle By Name(w139) -> ("Beam Type (-1/1)"=w133:dbl)
            n34 = Format Date/Time String(time format string (%c)="%H%M%S%3u", seconds (now)=w133) -> (date/time string=w134:string)  [unwired: 1 in]
            n35 = Concatenate Strings(w138, w134, w138) -> (w137:string)
            n36 = call "FITS - Format FITS Keyword v2 .vi"("Keyword"=w142, "Value"=w137, "Comment"=w141) -> ("Formatted fits entry"=w140:string, "Length of line"=w136:i16)  [unwired: 1 in, 1 out]
          }
          frame "ORIGIN" {
            w146 = "'" ("string")
            n37 = Concatenate Strings(w146, "AISAS", w146) -> (w145:string)
            n38 = call "FITS - Format FITS Keyword v2 .vi"("Keyword"=w149, "Value"=w145, "Comment"=w148) -> ("Formatted fits entry"=w147:string, "Length of line"=w143:i16)  [unwired: 1 in, 1 out]
          }
          frame "INSTRUME" {
            w153 = "'" ("string")
            n39 = disable-structure shown="SCMP==COMP, Default" {
              disable-tunnel: ["COMP-S" "SCD"] -> w151
              frame condition #0 (active) {
              }
              frame condition #1 {
              }
            }
            n40 = Concatenate Strings(w153, w151, w153) -> (w152:string)
            n41 = call "FITS - Format FITS Keyword v2 .vi"("Keyword"=w156, "Value"=w152, "Comment"=w155) -> ("Formatted fits entry"=w154:string, "Length of line"=w150:i16)  [unwired: 1 in, 1 out]
          }
          frame "TELESCOP" {
            w162 = "'" ("string")
            n42 = Concatenate Strings(w162, "20CM ZEISS", w162) -> (w160:string)
            n43 = call "FITS - Format FITS Keyword v2 .vi"("Keyword"=w165, "Value"=w160, "Comment"=w164) -> ("Formatted fits entry"=w163:string, "Length of line"=w159:i16)  [unwired: 1 in, 1 out]
          }
          frame "XTENSION" {
            n44 = call "FITS - Format FITS Keyword v2 .vi"("Keyword"=w170, "Value"="'IMAGE'", "Comment"=w169) -> ("Formatted fits entry"=w168:string, "Length of line"=w166:i16)  [unwired: 1 in, 1 out]
          }
          frame "PCOUNT" {
            n45 = call "FITS - Format FITS Keyword v2 .vi"("Keyword"=w175, "Value"="0", "Comment"=w173) -> ("Formatted fits entry"=w172:string, "Length of line"=w171:i16)  [unwired: 1 in, 1 out]
          }
          frame "GCOUNT" {
            n46 = call "FITS - Format FITS Keyword v2 .vi"("Keyword"=w180, "Value"="1", "Comment"=w178) -> ("Formatted fits entry"=w177:string, "Length of line"=w176:i16)  [unwired: 1 in, 1 out]
          }
          frame "LOCATION" {
            w185 = "'" ("string")
            n47 = Concatenate Strings(w185, "LOMNICKY PEAK OBS", w185) -> (w184:string)
            n48 = call "FITS - Format FITS Keyword v2 .vi"("Keyword"=w187, "Value"=w184, "Comment"=w182) -> ("Formatted fits entry"=w186:string, "Length of line"=w181:i16)  [unwired: 1 in, 1 out]
          }
          frame "TUNEDLAY" {
            n49 = Unbundle By Name(w189) -> ("Tuning Delay (ms)"=w195:dbl)
            n50 = Format Into String(format string="%0.3d", w195) -> (resulting string=w193:string)  [unwired: 2 in, 1 out]
            n51 = call "FITS - Format FITS Keyword v2 .vi"("Keyword"=w192, "Value"=w193, "Comment"=w191) -> ("Formatted fits entry"=w190:string, "Length of line"=w188:i16)  [unwired: 1 in, 1 out]
          }
          frame "FOCUS" {
            (unwired) "%0.3d" ("format string")
            n52 = Unbundle By Name(w198) -> ("Camera Position (mm)"=w197:dbl)
            n53 = Format Into String(w197) -> (resulting string=w202:string)  [unwired: 3 in, 1 out]
            n54 = call "FITS - Format FITS Keyword v2 .vi"("Keyword"=w201, "Value"=w202, "Comment"=w200) -> ("Formatted fits entry"=w199:string, "Length of line"=w196:i16)  [unwired: 1 in, 1 out]
          }
          frame "MODC" {
            n55 = Unbundle By Name(w205) -> ("Mod Cycles"=w204:u16)
            n56 = Format Into String(format string="%0.3d", w204) -> (resulting string=w209:string)  [unwired: 2 in, 1 out]
            n57 = call "FITS - Format FITS Keyword v2 .vi"("Keyword"=w208, "Value"=w209, "Comment"=w207) -> ("Formatted fits entry"=w206:string, "Length of line"=w203:i16)  [unwired: 1 in, 1 out]
          }
          frame "WAVELENG" {
            n58 = Unbundle By Name(w215) -> ("Wavelength (nm)"=w214:dbl)
            n59 = Format Into String(format string="%0.3f", w214) -> (resulting string=w212:string)  [unwired: 2 in, 1 out]
            n60 = call "FITS - Format FITS Keyword v2 .vi"("Keyword"=w218, "Value"=w212, "Comment"=w217) -> ("Formatted fits entry"=w216:string, "Length of line"=w211:i16)  [unwired: 1 in, 1 out]
          }
          frame "NLC-1" {
            n61 = Unbundle By Name(w225) -> ("Tuning Voltages"=w221:dbl[])
            n62 = Index Array(array=w221, index=0) -> (element=w220:dbl)
            n63 = Format Into String(format string="%0.3f", w220) -> (resulting string=w219:string)  [unwired: 2 in, 1 out]
            n64 = call "FITS - Format FITS Keyword v2 .vi"("Keyword"=w228, "Value"=w219, "Comment"=w227) -> ("Formatted fits entry"=w226:string, "Length of line"=w224:i16)  [unwired: 1 in, 1 out]
          }
          frame "NLC-2" {
            n65 = Unbundle By Name(w235) -> ("Tuning Voltages"=w231:dbl[])
            n66 = Index Array(array=w231, index=1) -> (element=w230:dbl)
            n67 = Format Into String(format string="%0.3f", w230) -> (resulting string=w229:string)  [unwired: 2 in, 1 out]
            n68 = call "FITS - Format FITS Keyword v2 .vi"("Keyword"=w238, "Value"=w229, "Comment"=w237) -> ("Formatted fits entry"=w236:string, "Length of line"=w234:i16)  [unwired: 1 in, 1 out]
          }
          frame "NLC-3" {
            n69 = Unbundle By Name(w245) -> ("Tuning Voltages"=w241:dbl[])
            n70 = Index Array(array=w241, index=2) -> (element=w240:dbl)
            n71 = Format Into String(format string="%0.3f", w240) -> (resulting string=w239:string)  [unwired: 2 in, 1 out]
            n72 = call "FITS - Format FITS Keyword v2 .vi"("Keyword"=w248, "Value"=w239, "Comment"=w247) -> ("Formatted fits entry"=w246:string, "Length of line"=w244:i16)  [unwired: 1 in, 1 out]
          }
          frame "NLC-4" {
            n73 = Unbundle By Name(w255) -> ("Tuning Voltages"=w251:dbl[])
            n74 = Index Array(array=w251, index=3) -> (element=w250:dbl)
            n75 = Format Into String(format string="%0.3f", w250) -> (resulting string=w249:string)  [unwired: 2 in, 1 out]
            n76 = call "FITS - Format FITS Keyword v2 .vi"("Keyword"=w258, "Value"=w249, "Comment"=w257) -> ("Formatted fits entry"=w256:string, "Length of line"=w254:i16)  [unwired: 1 in, 1 out]
          }
          frame "NLC-5" {
            n77 = Unbundle By Name(w265) -> ("Tuning Voltages"=w261:dbl[])
            n78 = Index Array(array=w261, index=4) -> (element=w260:dbl)
            n79 = Format Into String(format string="%0.3f", w260) -> (resulting string=w259:string)  [unwired: 2 in, 1 out]
            n80 = call "FITS - Format FITS Keyword v2 .vi"("Keyword"=w268, "Value"=w259, "Comment"=w267) -> ("Formatted fits entry"=w266:string, "Length of line"=w264:i16)  [unwired: 1 in, 1 out]
          }
          frame "CAM-SN1" {
            w271 = "'" ("string")
            n81 = Unbundle By Name(w273) -> ("Camera Serial Number"=w269:string[])
            n82 = Concatenate Strings(w271, w269, w271) -> (w270:string)
            n83 = call "FITS - Format FITS Keyword v2 .vi"("Keyword"=w276, "Value"=w270, "Comment"=w275) -> ("Formatted fits entry"=w274:string, "Length of line"=w272:i16)  [unwired: 1 in, 1 out]
          }
          frame "EXPOSURE" {
            n84 = Unbundle By Name(w280) -> ("Exposure (s)"=w278:dbl)
            n85 = Format Into String(w278) -> (resulting string=w279:string)  [unwired: 3 in, 1 out]
            n86 = call "FITS - Format FITS Keyword v2 .vi"("Keyword"=w283, "Value"=w279, "Comment"=w282) -> ("Formatted fits entry"=w281:string, "Length of line"=w277:i16)  [unwired: 1 in, 1 out]
          }
          frame "CAM-TEMP" {
            n87 = Unbundle By Name(w287) -> ("SCD Calibration Optics"=w285:T5)
            n88 = Format Into String(w285) -> (resulting string=w286:string)  [unwired: 3 in, 1 out]
            n89 = call "FITS - Format FITS Keyword v2 .vi"("Keyword"=w290, "Value"=w286, "Comment"=w289) -> ("Formatted fits entry"=w288:string, "Length of line"=w284:i16)  [unwired: 1 in, 1 out]
          }
          frame "BEAM" {
            n90 = Unbundle By Name(w294) -> ("Beam Type (-1/1)"=w292:dbl)
            n91 = Number To Decimal String(number=w292) -> (decimal integer string=w293:string)  [unwired: 1 out]
            n92 = call "FITS - Format FITS Keyword v2 .vi"("Keyword"=w297, "Value"=w293, "Comment"=w296) -> ("Formatted fits entry"=w295:string, "Length of line"=w291:i16)  [unwired: 1 in, 1 out]
          }
          frame "DIFFUSER" {
            w298 = "'" ("string")
            n93 = Unbundle By Name(w306) -> ("Light Shapping Diffuser"=w300:T4)
            n94 = Build Array("IN BEAM", "OUT OF BEAM") -> (w302:string[])
            n95 = Index Array(array=w302, index=w300) -> (element=w299:string)
            n96 = Concatenate Strings(w298, w299, w298) -> (w301:string)
            n97 = call "FITS - Format FITS Keyword v2 .vi"("Keyword"=w309, "Value"=w301, "Comment"=w308) -> ("Formatted fits entry"=w307:string, "Length of line"=w305:i16)  [unwired: 1 in, 1 out]
          }
          frame "FW-WVLNG" {
            w311 = "'" ("string")
            n98 = disable-structure shown="SCMP==COMP, Default" {
              disable-tunnel: w314 -> [w320 w334]
              disable-tunnel: [w318 w332] -> w310
              frame condition #0 {
                n99 = Unbundle By Name(w320) -> ("SCD Emission Line Filter"=w319:T6)
                n100 = Build Array("Not Used" ("element"), "557.6", "587.6", "589.6", "630.2", "656.4", "849.8", "854.2", "866.2", "1083.0") -> (w321:string[])
                n101 = Index Array(array=w321, index=w319) -> (element=w318:string)
              }
              frame condition #1 (active) {
                n102 = Unbundle By Name(w334) -> ("COMP-S Andover Filter Wheel"=w333:T8)
                n103 = Build Array("Not Used" ("element"), "530,3", "587.6", "637,5", "656,3", "789,2", "854,2", "1074,7", "1079,8", "1083.0") -> (w335:string[])
                n104 = Index Array(array=w335, index=w333) -> (element=w332:string)
              }
            }
            n105 = Concatenate Strings(w311, w310, w311) -> (w312:string)
            n106 = call "FITS - Format FITS Keyword v2 .vi"("Keyword"=w317, "Value"=w312, "Comment"=w316) -> ("Formatted fits entry"=w315:string, "Length of line"=w313:i16)  [unwired: 1 in, 1 out]
          }
          frame "FW-CALIB" {
            w346 = "'" ("string")
            n107 = disable-structure shown="SCMP==COMP, Default" {
              disable-tunnel: w350 -> [w367 w381]
              disable-tunnel: [w365 w379] -> w347
              frame condition #0 {
                n108 = Unbundle By Name(w367) -> ("SCD Calibration Optics"=w366:T5)
                n109 = Build Array("Not Used" ("element"), "LP0, I+Q", "LP90, I-Q", "LP45, I+U", "LP135, I-U" ("element"), "LCP, I+V" ("element"), "RCP, I-V" ("element"), "Dark" ("element"), "Clear" ("element"), "N/A" ("element")) -> (w354:string[])
                n110 = Index Array(array=w354, index=w366) -> (element=w365:string)
              }
              frame condition #1 (active) {
                n111 = Unbundle By Name(w381) -> ("COMP-S Calibration Wheel"=w380:T7)
                n112 = Build Array("Not Used" ("element"), "Dark", "Clear", "Lens", "I+Q" ("element"), "I-Q" ("element"), "I+U" ("element"), "I-U" ("element"), "I+V" ("element"), "I-V" ("element")) -> (w370:string[])
                n113 = Index Array(array=w370, index=w380) -> (element=w379:string)
              }
            }
            n114 = Concatenate Strings(w346, w347, w346) -> (w348:string)
            n115 = call "FITS - Format FITS Keyword v2 .vi"("Keyword"=w353, "Value"=w348, "Comment"=w352) -> ("Formatted fits entry"=w351:string, "Length of line"=w349:i16)  [unwired: 1 in, 1 out]
          }
          frame "ROTPOS" {
            n116 = Unbundle By Name(w389) -> ("FOV Rotation (deg)"=w388:dbl)
            n117 = Format Into String(format string="%0.1f", w388) -> (resulting string=w387:string)  [unwired: 2 in, 1 out]
            n118 = call "FITS - Format FITS Keyword v2 .vi"("Keyword"=w385, "Value"=w387, "Comment"=w386) -> ("Formatted fits entry"=w384:string, "Length of line"=w383:i16)  [unwired: 1 in, 1 out]
          }
          frame "BSCALE" {
            n119 = call "FITS - Format FITS Keyword v2 .vi"("Keyword"=w394, "Value"="1.", "Comment"=w393) -> ("Formatted fits entry"=w392:string, "Length of line"=w391:i16)  [unwired: 1 in, 1 out]
          }
          frame "BZERO" {
            (unwired) "32768." ("Value")
            n120 = call "FITS - Format FITS Keyword v2 .vi"("Keyword"=w399, "Value"="BZERO", "Comment"=w398) -> ("Formatted fits entry"=w397:string, "Length of line"=w396:i16)  [unwired: 1 in, 1 out]
          }
          frame "COOKBOOK" {
            n121 = Unbundle By Name(w405) -> ("Cookbook"=w400:string)
            n122 = call "FITS - Format FITS Keyword v2 .vi"("Keyword"=w404, "Value"=w400, "Comment"=w403) -> ("Formatted fits entry"=w402:string, "Length of line"=w401:i16)  [unwired: 1 in, 1 out]
          }
          frame "DATATYPE" {
            (unwired) u16 9 items=["DARK", "FLAT", "CALI", "OBSE", "ABSO", "AURE", "TARG", "OBJE", "HOLE", "LIVE"] ("Data Type")
            n123 = Unbundle By Name(w412) -> ("Data Type"=w407:u16)
            n124 = case shown="9" w407 {
              tunnel: ["DARK" "FLAT" "CALI" "OBSE" "ABSO" "AURE" "TARG" "OBJE" "HOLE" "LIVE"] -> w406
              frame 0, Default {
              }
              frame 1 {
              }
              frame 2 {
              }
              frame 3 {
              }
              frame 4 {
              }
              frame 5 {
              }
              frame 6 {
              }
              frame 7 {
              }
              frame 8 {
              }
              frame 9 {
              }
            }
            n125 = call "FITS - Format FITS Keyword v2 .vi"("Keyword"=w411, "Value"=w406, "Comment"=w410) -> ("Formatted fits entry"=w409:string, "Length of line"=w408:i16)  [unwired: 1 in, 1 out]
          }
        }
      }
      n126 = Array Size(array=w11) -> (size(s)=w6:i32)
      "Header Rows" <- w6
      n127 = Divide(x=23040, y=80) -> (x/y=w7:dbl)
      n128 = Subtract(x=w7, y=w6) -> (x-y=w5:dbl)
      n129 = Decrement(x=w5) -> (x-1=w4:dbl)
      "Required COMMENT Rows" <- w4
      n130 = Format Into String(format string="COMMENT%73s", "") -> (resulting string=w14:string)  [unwired: 2 in, 1 out]
      n131 = for {
        N: w4 -> [_]
        tunnel: w14 -> [w32]
        tunnel: [w32] -> w13 mode=indexing
      }
      n132 = Format Into String(format string="END%77s", "") -> (resulting string=w18:string)  [unwired: 2 in, 1 out]
      n133 = Build Array (concatenate)(w11, w13, w18) -> (w20:string[])
      "FITS Header" <- w20
      n134 = for {
        tunnel: w20 -> [w34] mode=indexing
        shift-right: [w35] -> w17
        shift-left: "" -> [w33]
        n135 = Concatenate Strings(w33, w34) -> (w35:string)
      }
      "23040 Byte Header" <- w17
      n136 = String Length(string=w17) -> (length=→"final header byte length":i32)
    }
    frame Error {
    }
  }
  "error out" <- w1
